vi "Find Event Frame.vi"(8 "error in":errorcluster, 9 "VI":refnum<class "VI.lvclass">, 10 "Library":refnum<class "Library.lvclass">, 11 "Project":refnum<class "Project.lvclass">) -> (0 "error out":errorcluster)   [LabVIEW 2020, in "Panther Dashboard.lvlib"]
uses:
  Panther Dashboard.lvlib
  Class/VI/VI.lvclass
  C:/GitClones/PantherDashboard/src/LabVIEW/Panther Dashboard/Class/LabVIEWItem/LabVIEWItem.lvclass
  Class/Library/Library.lvclass
  Class/Project/Project.lvclass
  Class/LabVIEWItem/Item Type--enum.ctl
  Class/LabVIEWItem/LabVIEWItem.lvclass/LabVIEWItem.ctl
  Class/Project/Project.lvclass/Project.ctl
  19d5df14-f93c-4814-961c-bd3574541912.vi
  Class/LabVIEWItem/Read Item Name.vi
  Class/LabVIEWItem/Read Item Path.vi
  Class/LabVIEWItem/Read Item Type.vi
  Class/Project/Read Main App Inst Ref.vi
  Class/LabVIEWItem/LabVIEWItem.lvclass
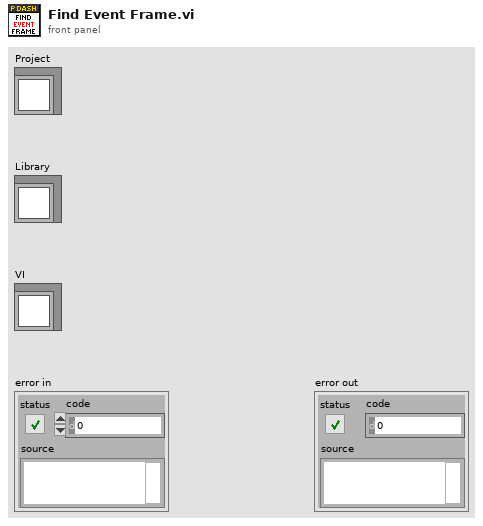
[diagram p1: front panel]
types:
  T1 = typedef "Panther Dashboard.lvlib/LabVIEWItem.lvclass/Item Type--enum.ctl" = enum16{"Requests", "Broadcasts", "Request and Wait for Reply", "Round Trip", "» Public API VIs", "» Constant VIs", "» Error VIs", "Module", "Project", "No Drag Selection"}
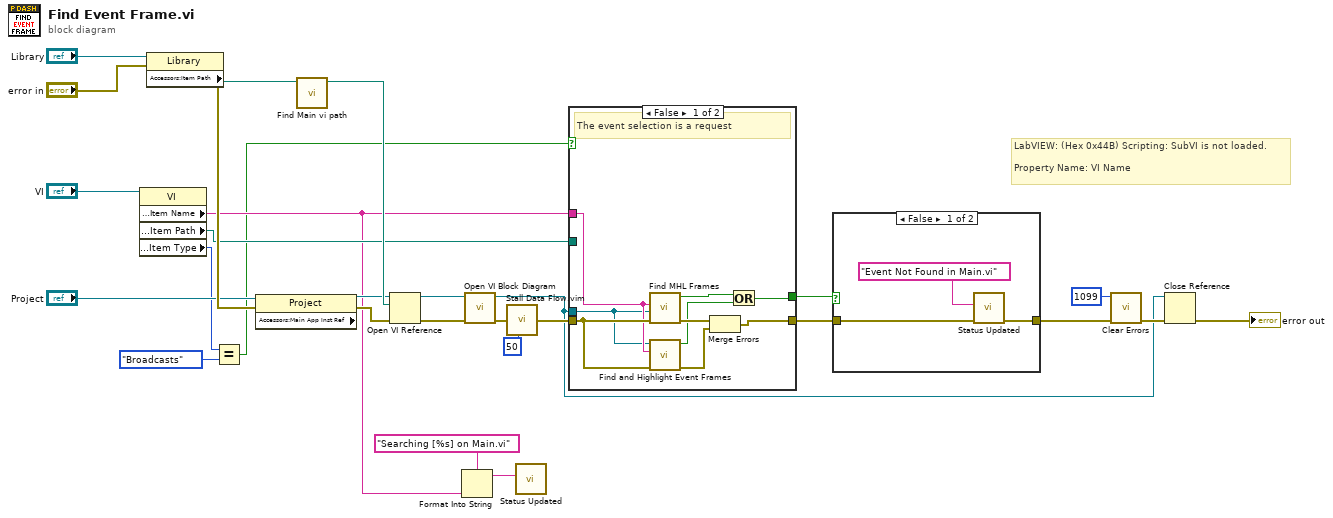
[diagram p0: block diagram]
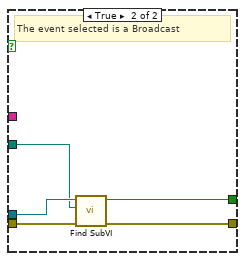
[diagram p3: hidden frame]
diagram:
  # "LabVIEW: (Hex 0x44B) Scripting: SubVI is not loaded.\n\nProperty Name: VI Name"
  n1 = property class="VI"(reference="VI") -> ("Accessors:Item Name"=w4:string, "Accessors:Item Path"=w5:path, "Accessors:Item Type"=w3:T1)  [unwired: 1 in, 2 out]
  n2 = property class="Library"(reference="Library", error in="error in") -> (error out=w20:errorcluster, "Accessors:Item Path"=w10:path)  [unwired: 1 out]
  n3 = Equal?(x=w3, y=Item_Type--enum."Broadcasts") -> (x = y?=w1:bool)
  n4 = property class="Project"(reference="Project", error in=w20) -> (error out=w21:errorcluster, "Accessors:Main App Inst Ref"=w7:refnum<vi>)  [unwired: 1 out]
  n5 = call "Find Main vi path.vi"("Library Path"=w10) -> ("Main vi Path"=w9:path)  [unwired: 10 in]
  n6 = Open VI Reference(application reference (local)=w7, vi path=w9, error in (no error)=w21) -> (vi reference=w15:refnum<vi>, error out=w26:errorcluster)  [unwired: 3 in]
  n7 = Format Into String(format string="Searching [%s] on Main.vi", w4) -> (resulting string=w18:string)  [unwired: 2 in, 1 out]
  n8 = call "Open VI Block Diagram.vi"("error in (no error)"=w26, "VI in"=w15) -> ("error out"=w27:errorcluster, "VI out"=w14:refnum<vi>)  [unwired: 8 in]
  n9 = call "Stall Data Flow.vim"("value in"=w27, "milliseconds to wait"=u32 50) -> ("value out"=w25:errorcluster)  [unwired: 1 out]
  n10 = call "Status Updated.vi"("Status"=w18) -> ()  [unwired: 10 in, 1 out]
  n11 = case shown="False" w1 {
    tunnel: w25 -> [w37 w42]
    tunnel: w4 -> [w33 _]
    tunnel: [w34 w41] -> w23
    tunnel: w14 -> [w32 w40]
    tunnel: [w29 w39] -> w12
    tunnel: w5 -> [_ w38]
    frame False {
      # "The event selection is a request"
      n12 = call "Find MHL Frames.vi"("error in"=w37, "Event Name"=w33, "VI reference"=w32) -> ("error out"=w36:errorcluster, "Found?"=w30:bool)  [unwired: 7 in]
      n13 = call "Find and Highlight Event Frames.vi"("error in"=w37, "Event Name"=w33, "VI Reference"=w32) -> ("error out"=w35:errorcluster, "Found?"=w31:bool)  [unwired: 7 in]
      n14 = Merge Errors(w36, w35) -> (w34:errorcluster)
      n15 = Or(x=w30, y=w31) -> (x .or. y?=w29:bool)
    }
    frame True {
      # "The event selected is a Broadcast"
      n16 = call "Find SubVI.vi"("error in"=w42, "VI Path"=w38, "VI Reference"=w40) -> ("error out"=w41:errorcluster, "Found?"=w39:bool)  [unwired: 7 in]
    }
  }
  n17 = case shown="False" w12 {
    tunnel: w23 -> [w45 w46]
    tunnel: [w44 w46] -> w22
    frame False {
      n18 = call "Status Updated.vi"("error in (no error)"=w45, "Status"="Event Not Found in Main.vi") -> ("error out"=w44:errorcluster)  [unwired: 9 in]
    }
    frame True {
      # "Found Event"
    }
  }
  n19 = call <vilib>:"Clear Errors.vi"("error in (no error)"=w22, "specific error code to clear (0: all)"=1099) -> ("error out"=w28:errorcluster)  [unwired: 4 in, 1 out]
  n20 = Close Reference(reference=w14, error in (no error)=w28) -> (error out=→"error out":errorcluster)
